vi "打包属性.vi"(4 "样品标记":string, 6 "测试参数":variant, 7 "循环":bool, 8 "错误输入":errorcluster, 11 "功能":string) -> (0 "错误输出":errorcluster, 3 "数据属性":variant)   [LabVIEW 2020]
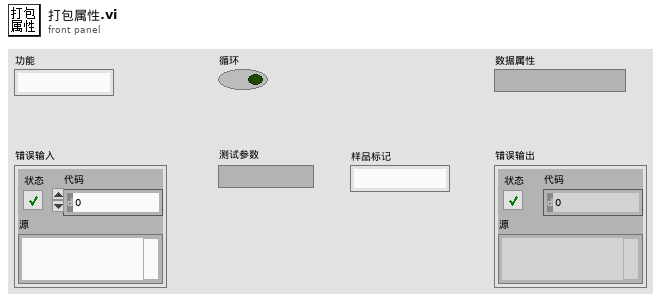
[diagram p1: front panel]
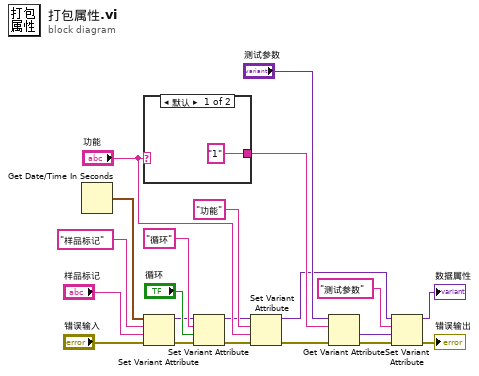
[diagram p0: block diagram]
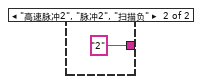
[diagram p2: hidden frame]
diagram:
  n1 = Get Date/Time In Seconds() -> (seconds since 1Jan1904=w1:timestamp)
  n2 = case shown="默认" "功能" {
    tunnel: ["1" ("名称") "2" ("名称")] -> w11
    frame Default {
    }
    frame "高速脉冲2", "脉冲2", "扫描负" {
    }
  }
  n3 = Set Variant Attribute(Variant=w1, name="样品标记" ("元素"), value="样品标记", error in="错误输入") -> (Variant out=w7:variant, error out=w6:errorcluster)  [unwired: 1 out]
  n4 = Set Variant Attribute(Variant=w7, name="循环" ("元素"), value="循环", error in=w6) -> (Variant out=w5:variant, error out=w4:errorcluster)  [unwired: 1 out]
  n5 = Set Variant Attribute(Variant=w5, name="功能" ("元素"), value="功能", error in=w4) -> (Variant out=w2:variant, error out=w3:errorcluster)  [unwired: 1 out]
  n6 = Get Variant Attribute(Variant="测试参数", name=w11, error in=w3) -> (value=w8:variant, error out=w9:errorcluster)  [unwired: 1 in, 2 out]
  n7 = Set Variant Attribute(Variant=w2, name="测试参数" ("元素"), value=w8, error in=w9) -> (Variant out=→"数据属性":variant, error out=→"错误输出":errorcluster)  [unwired: 1 out]
